vi "Set-ConstantOutput.vi"(4 "error in (no error)":errorcluster, 5 "Voltage / Volts":dbl min=-15.0 max=15.0, 6 "Output channel":T1, 7 "VISA resource name":refnum<visa-resource-name>="COM7") -> (0 "error out":errorcluster={"status"=TRUE, "code"=10, "source"="Setting the limits failed: return values not echoed correctly."}, 1 "VISA resource name out":refnum<visa-resource-name>="COM7")   [LabVIEW 2015, in "YbTempCtrl.lvlib"]
doc: "<B>DANGER: THIS VI CAN BLOW THINGS UP!</B>\nOutput a constant voltage on the given channel. Positive and negative numbers accepted.\nInput should be scaled from -1 to +1"
uses:
  YbTempCtrl.lvlib
  Typedefs/OutputChannelTypedef.ctl
panel:
  out "Output Str":string
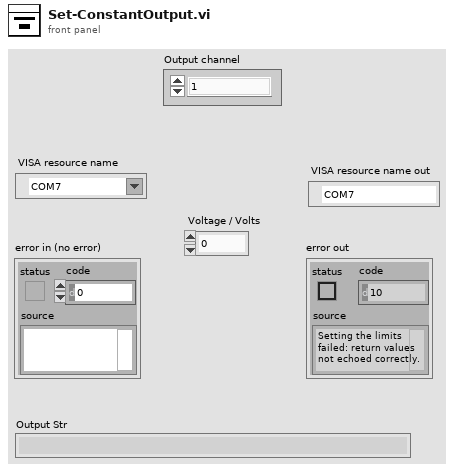
[diagram p1: front panel]
types:
  T1 = typedef "YbTempCtrl.lvlib/OutputChannelTypedef.ctl" = enum16{"1", "2", "3", "4", "BPA", "BPB"}
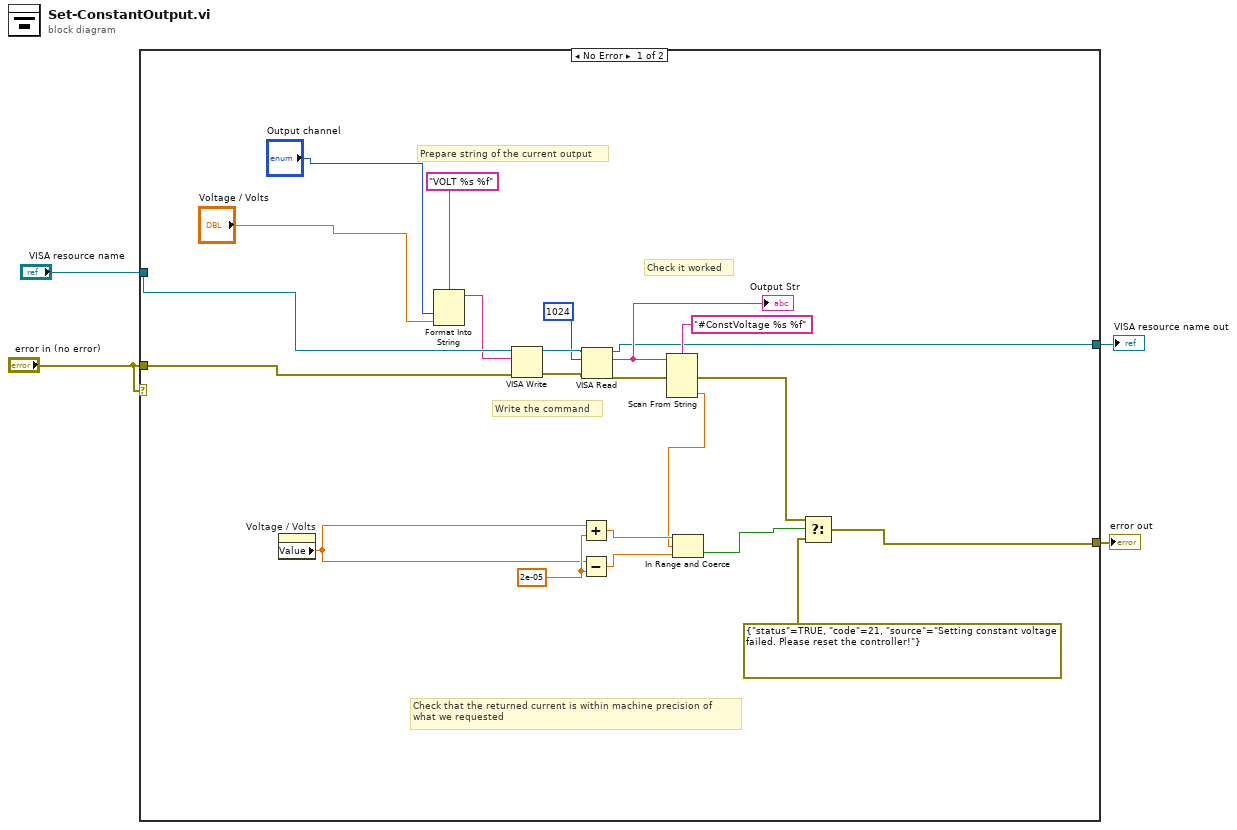
[diagram p0: block diagram]
diagram:
  n1 = case shown="No Error" "error in (no error)" {
    tunnel: "VISA resource name" -> [w11 w27]
    tunnel: "error in (no error)" -> [w10 w28]
    tunnel: [w14 w27] -> w3
    tunnel: [w13 w28] -> w2
    frame No Error {
      w25 = 2e-05
      # "Check that the returned current is within machine precision of\nwhat we requested"
      # "Check it worked"
      # "Write the command"
      # "Prepare string of the current output"
      n2 = property on="Voltage / Volts" class="DigNum (strict)"() -> ("Value"=w7:dbl)  [unwired: 2 in, 2 out]
      n3 = Format Into String(format string="VOLT %s %f", "Output channel", "Voltage / Volts") -> (resulting string=w9:string)  [unwired: 2 in, 1 out]
      n4 = VISA Write(VISA resource name=w11, write buffer=w9, error in (no error)=w10) -> (VISA resource name out=w21:refnum<visa-resource-name>, error out=w20:errorcluster)  [unwired: 1 out]
      n5 = Add(x=w7, y=w25) -> (x+y=w24:dbl)
      n6 = Subtract(x=w7, y=w25) -> (x-y=w23:dbl)
      n7 = VISA Read(VISA resource name=w21, byte count=u32 1024, error in (no error)=w20) -> (VISA resource name out=w14:refnum<visa-resource-name>, read buffer=w18:string, error out=w17:errorcluster)  [unwired: 1 out]
      "Output Str" <- w18
      n8 = Scan From String(format string="#ConstVoltage %s %f", input string=w18, error in=w17) -> (error out=w16:errorcluster, output 2=w12:dbl)  [unwired: 4 in, 2 out]
      n9 = In Range and Coerce(upper limit=w24, x=w12, lower limit=w23) -> (In Range?=w6:bool)  [unwired: 1 out]
      n10 = Select(t=w16, s=w6, f=errorcluster {"status"=TRUE, "code"=21, "source"="Setting constant voltage failed. Please reset the controller!"}) -> (s? t:f=w13:errorcluster)
    }
    frame Error {
    }
  }
  "VISA resource name out" <- w3
  "error out" <- w2
